vi "LoopVI.vi"() -> ()   [LabVIEW 2013]
uses:
  <vilib>/Utility/file.llb/Read From Spreadsheet File (DBL).vi
panel:
  in  "Boolean":bool
  in  "measurement file\n\n         ??. txt":bool
  out "free gas model":cluster{"Y":dbl[], "Y":dbl[]}[](graph)
  in  "Fermi angle\n   (mrad)":dbl=7.0
  in  "stop 2":bool
  out "core electrons":cluster{"Y":dbl[], "Y":dbl[]}[](graph)
  in  "core width\n   (mrad)":dbl=5.0
  in  "fraction core\nannihilations":dbl=0.2 min=0.0 max=1.0 step=1e-05
  out "ZICHT  functie":cluster{"Y":dbl[], "Y":dbl[]}[](graph)
  in  "spleetbreedte\n      (mm)":dbl=1.0 min=0.1 max=5.0
  in  "collimator afstand\n       (mm)":dbl=500.0 min=100.0 max=1000.0
  in  "stop 4":bool
  out "XY Graph 4":cluster{ext[], "Array out":ext[]}[](graph)
  in  "alignment correction":dbl min=-10.0 max=10.0 step=0.0001
  in  "background \n coincidence counts":dbl min=0.0 max=100.0
  out "Fermi energy (eV)":dbl format="%#_3g"
  in  "22Na source radius (mm)":dbl=0.1 min=1e-05 max=3.0
  out "?":dbl format="%#_3g"
  in  "1d - Acar":bool caption="2d - Acar or DB"
  out "2d - Acar 2":bool
  out "2d - Acar 3":bool
  out "2d - Acar 4":bool
  out "XY Graph 5":cluster{ext[], "Array out":ext[]}[](graph)
  out "output cluster 2":cluster{ext[], ext[]}
  out "Sum of squared residuals":dbl
  in  "sigma (mrad) 2":dbl
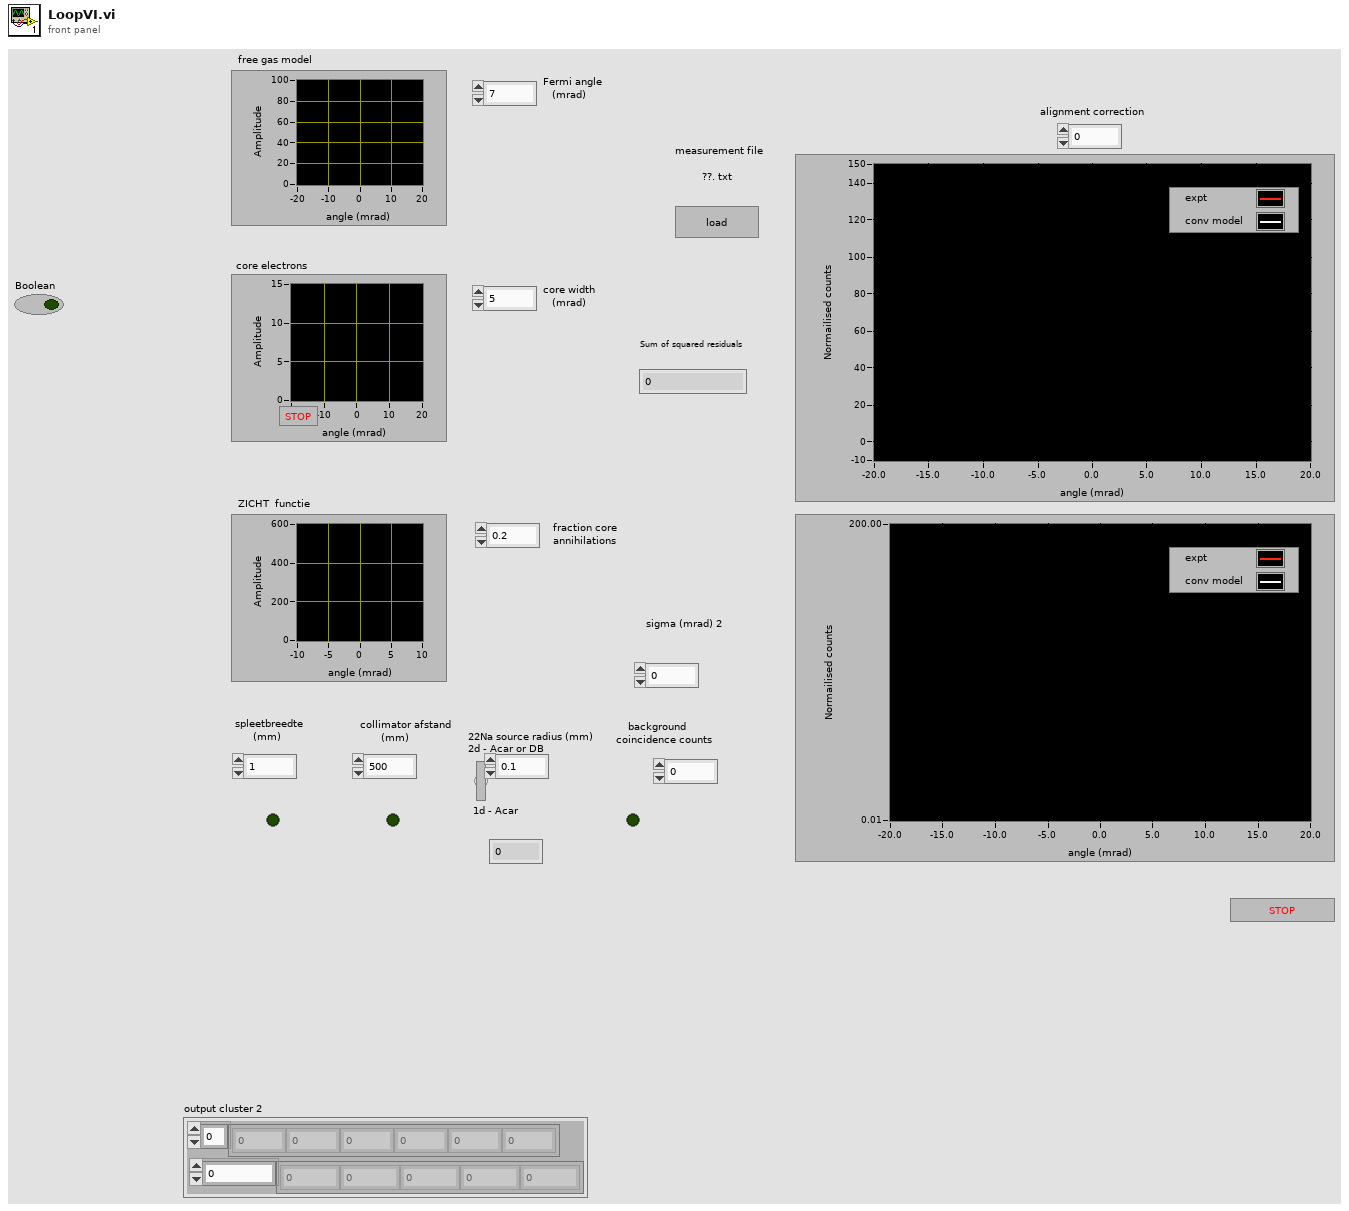
[diagram p1: front panel]
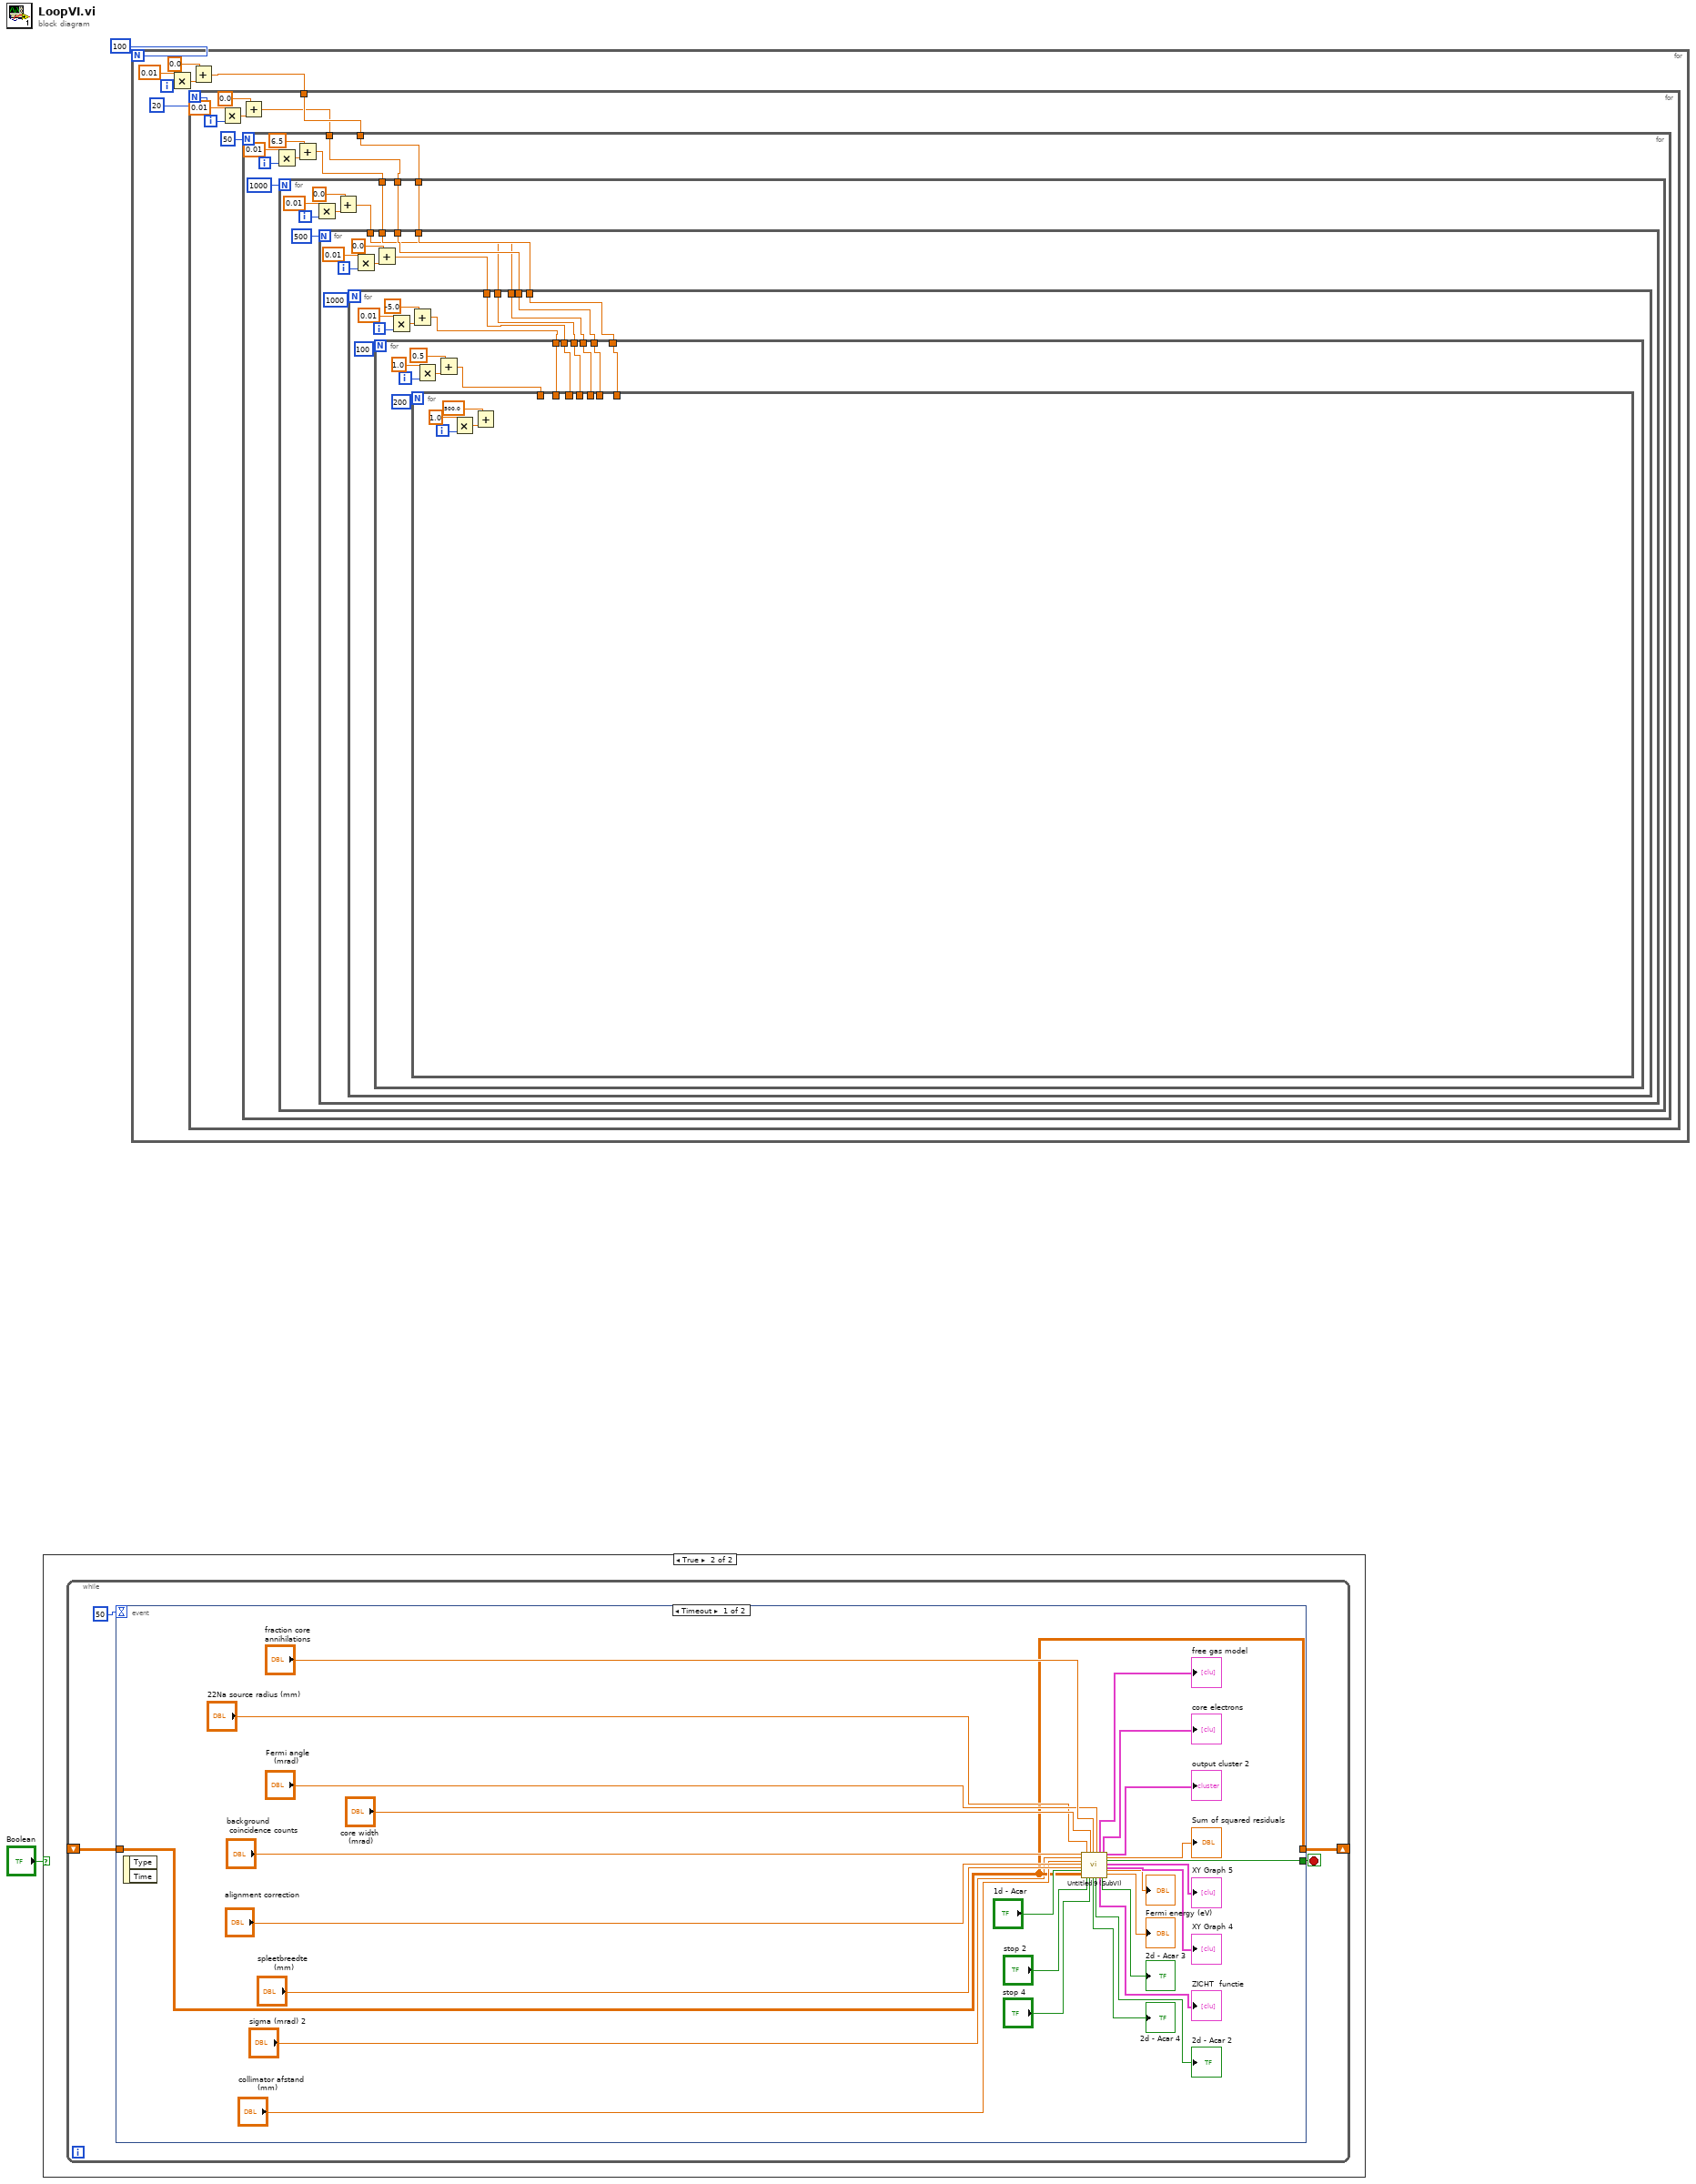
[diagram p0: block diagram]
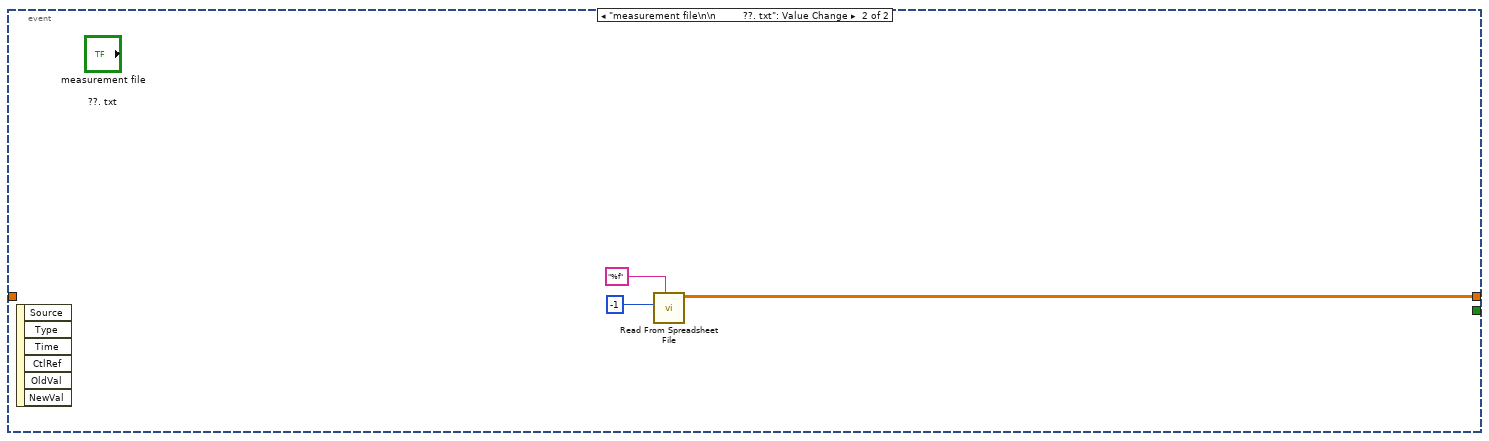
[diagram p3: hidden frame]
diagram:
  n1 = case shown="True" "Boolean" {
    frame False {
    }
    frame True {
      n2 = while {
        shift-right: [w4] -> _
        shift-left: _ -> [w3]
        stop <- w6 stop-if-true
        n3 = event shown="[0] Timeout" {
          selector: _ -> [_ _]
          dyn-events: _ -> [_ _]
          timeout: 50 -> [_ _]
          tunnel: [w32 _] -> w6
          tunnel: [w22 w34] -> w4
          tunnel: w3 -> [w22 _]
          event Timeout {
            n4 = event-data() -> ()  [unwired: 1 in, 2 out]
            n5 = call "Untitled 9 (SubVI).vi"("background \n coincidence counts"="background \n coincidence counts", "sigma (mrad) in"="sigma (mrad) 2", "collimator afstand\n       (mm)"="collimator afstand\n       (mm)", "alignment correction"="alignment correction", "spleetbreedte\n      (mm)"="spleetbreedte\n      (mm)", "1d - Acar"="1d - Acar", "all rows"=w22, "22Na source radius (mm)"="22Na source radius (mm)", "stop in"="stop 2", "core width\n   (mrad)"="core width\n   (mrad)", "stop 4"="stop 4", "fraction core\nannihilations"="fraction core\nannihilations", "Fermi angle\n   (mrad)"="Fermi angle\n   (mrad)") -> ("2d - Acar 4"=→"2d - Acar 4":bool, "2d - Acar 2"=→"2d - Acar 2":bool, "free gas model"=→"free gas model":cluster{"Y":dbl[], "Y":dbl[]}[], "ZICHT  functie"=→"ZICHT  functie":cluster{"Y":dbl[], "Y":dbl[]}[], "core electrons"=→"core electrons":cluster{"Y":dbl[], "Y":dbl[]}[], "2d - Acar 3"=→"2d - Acar 3":bool, "output cluster 2"=→"output cluster 2":cluster{ext[], ext[]}, "Sum of squared residuals"=→"Sum of squared residuals":dbl, "stop 3"=w32:bool, "XY Graph 5"=→"XY Graph 5":cluster{ext[], "Array out":ext[]}[], "XY Graph 4"=→"XY Graph 4":cluster{ext[], "Array out":ext[]}[], 25:→"?":dbl, "Fermi energy (eV)"=→"Fermi energy (eV)":dbl)  [unwired: 2 in]
          }
          event "measurement file\n\n         ??. txt": Value Change {
            n6 = event-data() -> ()  [unwired: 1 in, 6 out]
            n7 = call-poly <vilib>:"Read From Spreadsheet File.vi"("format (%.3f)"="%f", "number of rows (all:-1)"=-1) -> ("all rows"=w34:ext[][])  [unwired: 5 in, 4 out]
          }
        }
      }
    }
  }
  n8 = for {
    N: 100 -> [_]
    i -> [w41]
    n9 = Multiply(x=0.01, y=w41) -> (x*y=w39:dbl)
    n10 = Add(x=0.0, y=w39) -> (x+y=w37:dbl)
    n11 = for {
      N: 20 -> [_]
      tunnel: w37 -> [w43]
      i -> [w48]
      n12 = Multiply(x=0.01, y=w48) -> (x*y=w46:dbl)
      n13 = Add(x=0.0, y=w46) -> (x+y=w42:dbl)
      n14 = for {
        N: 50 -> [_]
        tunnel: w43 -> [w51]
        tunnel: w42 -> [w50]
        i -> [w56]
        n15 = Multiply(x=0.01, y=w56) -> (x*y=w54:dbl)
        n16 = Add(x=6.5, y=w54) -> (x+y=w49:dbl)
        n17 = for {
          N: 1000 -> [_]
          tunnel: w51 -> [w57]
          tunnel: w50 -> [w58]
          tunnel: w49 -> [w59]
          i -> [w65]
          n18 = Multiply(x=0.01, y=w65) -> (x*y=w63:dbl)
          n19 = Add(x=0.0, y=w63) -> (x+y=w60:dbl)
          n20 = for {
            N: 500 -> [_]
            tunnel: w60 -> [w67]
            tunnel: w59 -> [w68]
            tunnel: w58 -> [w69]
            tunnel: w57 -> [w70]
            i -> [w75]
            n21 = Multiply(x=0.01, y=w75) -> (x*y=w73:dbl)
            n22 = Add(x=0.0, y=w73) -> (x+y=w66:dbl)
            n23 = for {
              N: 1000 -> [_]
              tunnel: w70 -> [w81]
              tunnel: w69 -> [w80]
              tunnel: w68 -> [w79]
              tunnel: w67 -> [w78]
              tunnel: w66 -> [w77]
              i -> [w86]
              n24 = Multiply(x=0.01, y=w86) -> (x*y=w84:dbl)
              n25 = Add(x=-5.0, y=w84) -> (x+y=w76:dbl)
              n26 = for {
                N: 100 -> [_]
                tunnel: w81 -> [w92]
                tunnel: w80 -> [w91]
                tunnel: w79 -> [w90]
                tunnel: w78 -> [w89]
                tunnel: w77 -> [w88]
                tunnel: w76 -> [w87]
                i -> [w98]
                n27 = Multiply(x=1.0, y=w98) -> (x*y=w96:dbl)
                n28 = Add(x=0.5, y=w96) -> (x+y=w93:dbl)
                n29 = for {
                  N: 200 -> [_]
                  tunnel: w93 -> [_]
                  tunnel: w92 -> [_]
                  tunnel: w91 -> [_]
                  tunnel: w90 -> [_]
                  tunnel: w89 -> [_]
                  tunnel: w88 -> [_]
                  tunnel: w87 -> [_]
                  i -> [w102]
                  n30 = Multiply(x=1.0, y=w102) -> (x*y=w100:dbl)
                  n31 = Add(x=500.0, y=w100) -> ()  [unwired: 1 out]
                }
              }
            }
          }
        }
      }
    }
  }
